vi "Relink.vi"(0 "Parallel in":refnum<class "Parallel.lvclass">, 1 "Linked List Ref":refnum<data-value>, 2 "File Path":path, 5 "Flattened Test Executive":string, 7 "Return":string, 9 "Linked List ID":string, 11 "error in (no error)":errorcluster, 12 "Persistence in":refnum<class "IPersist.lvclass">, 13 "Compatibility Helper":refnum<class "ICompatibility Helper.lvclass">, 14 "Path Builder":refnum<class "IPath Builder.lvclass">) -> (3 "Linked List Ref out":refnum<data-value>, 6 "Flattened Test Executive out":string, 8 "Return out":string, 15 "error out":errorcluster)   [LabVIEW 2019, in "Test Executive.lvlib" / "Parallel.lvclass"]
uses:
  <vilib>/gpm_packages/@cs/test-executive/Source/Test Executive/Parallel/Parallel.lvclass
  <vilib>/gpm_packages/@cs/persistence/source/IPersist/IPersist.lvclass
  <vilib>/gpm_packages/@cs/linked-list/Source/Linked List/ILinkedList/ILinked List.lvclass
  <vilib>/gpm_packages/@cs/test-executive/Source/Path Builder/IPath Builder/IPath Builder.lvclass
  <vilib>/gpm_packages/@cs/test-executive/Source/Compatibility Helper/ICompatibility Helper.lvclass
  <vilib>/gpm_packages/@cs/test-executive/Source/Test Executive/Executioner/Executioner.lvclass
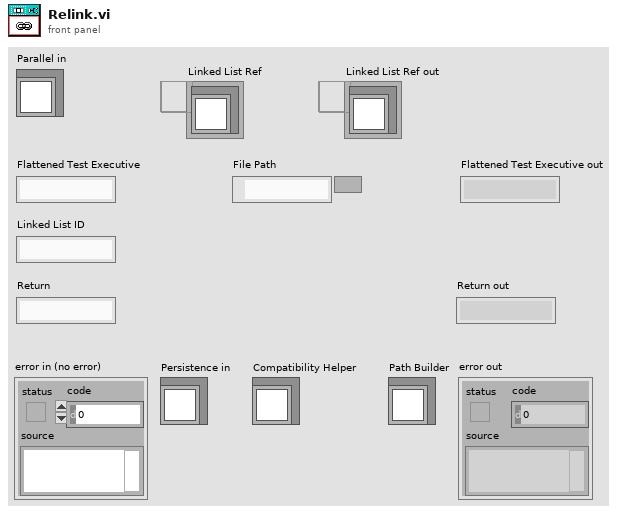
[diagram p1: front panel]
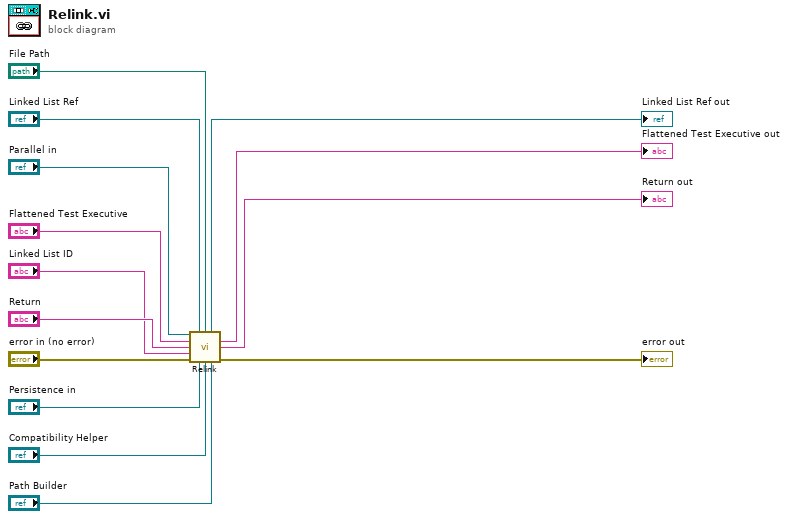
[diagram p0: block diagram]
diagram:
  n1 = call-parent "Relink.vi"("Executioner in"="Parallel in", "Linked List Ref"="Linked List Ref", "File Path"="File Path", "Flattened Test Executive"="Flattened Test Executive", "Return"="Return", "Linked List ID"="Linked List ID", "error in (no error)"="error in (no error)", "Persistence in"="Persistence in", "Compatibility Helper"="Compatibility Helper", "Path Builder"="Path Builder") -> ("Linked List Ref out"=→"Linked List Ref out":refnum<data-value>, "Flattened Test Executive out"=→"Flattened Test Executive out":string, "Return out"=→"Return out":string, "error out"=→"error out":errorcluster)  [unwired: 2 in]
